vi "Individual curve visualization.vi"() -> ()   [LabVIEW 2020]
uses:
  <vilib>/Analysis/NI_AALPro.lvlib
panel:
  in  "parameter bounds":T1={"amp min"=-inf, "amp max"=inf, "power min"=-inf, "power max"=inf, "offset min"=0.0, "offset max"=0.0}
  out "residue":dbl
  out "amplitude":dbl
  out "Fitoffset":dbl
  out "power":dbl
  in  "Tab Control":enum32{"Drag R and 4T R", " Line cut"}(tab)=enum." Line cut"
  in  "Input figure":cluster{dbl[], dbl[]}[](graph)
  out "Mean vs Curve":cluster{dbl[], dbl[]}(graph)
  in  "Group #":i32=40
  out "Power vs Cursorx":cluster{dbl[], dbl[]}(graph)
  out "Waveform Chart":T2(graph)={"Cursor.Cursor Y"=229.6975806451613, "Cursor.Cursor X"=-46.37419354838706}
  in  "Drag V from V2":dbl[][](graph)=array2400x360[864000 elements]
  out "Vcut":cluster{dbl[], "Best Power Fit":dbl[]}[](graph)
  out "Idrive":cluster{dbl[], dbl[]}[](graph)
  out "Residue of T vs Cursorx":cluster{dbl[], dbl[]}(graph)
  in  "stop":bool
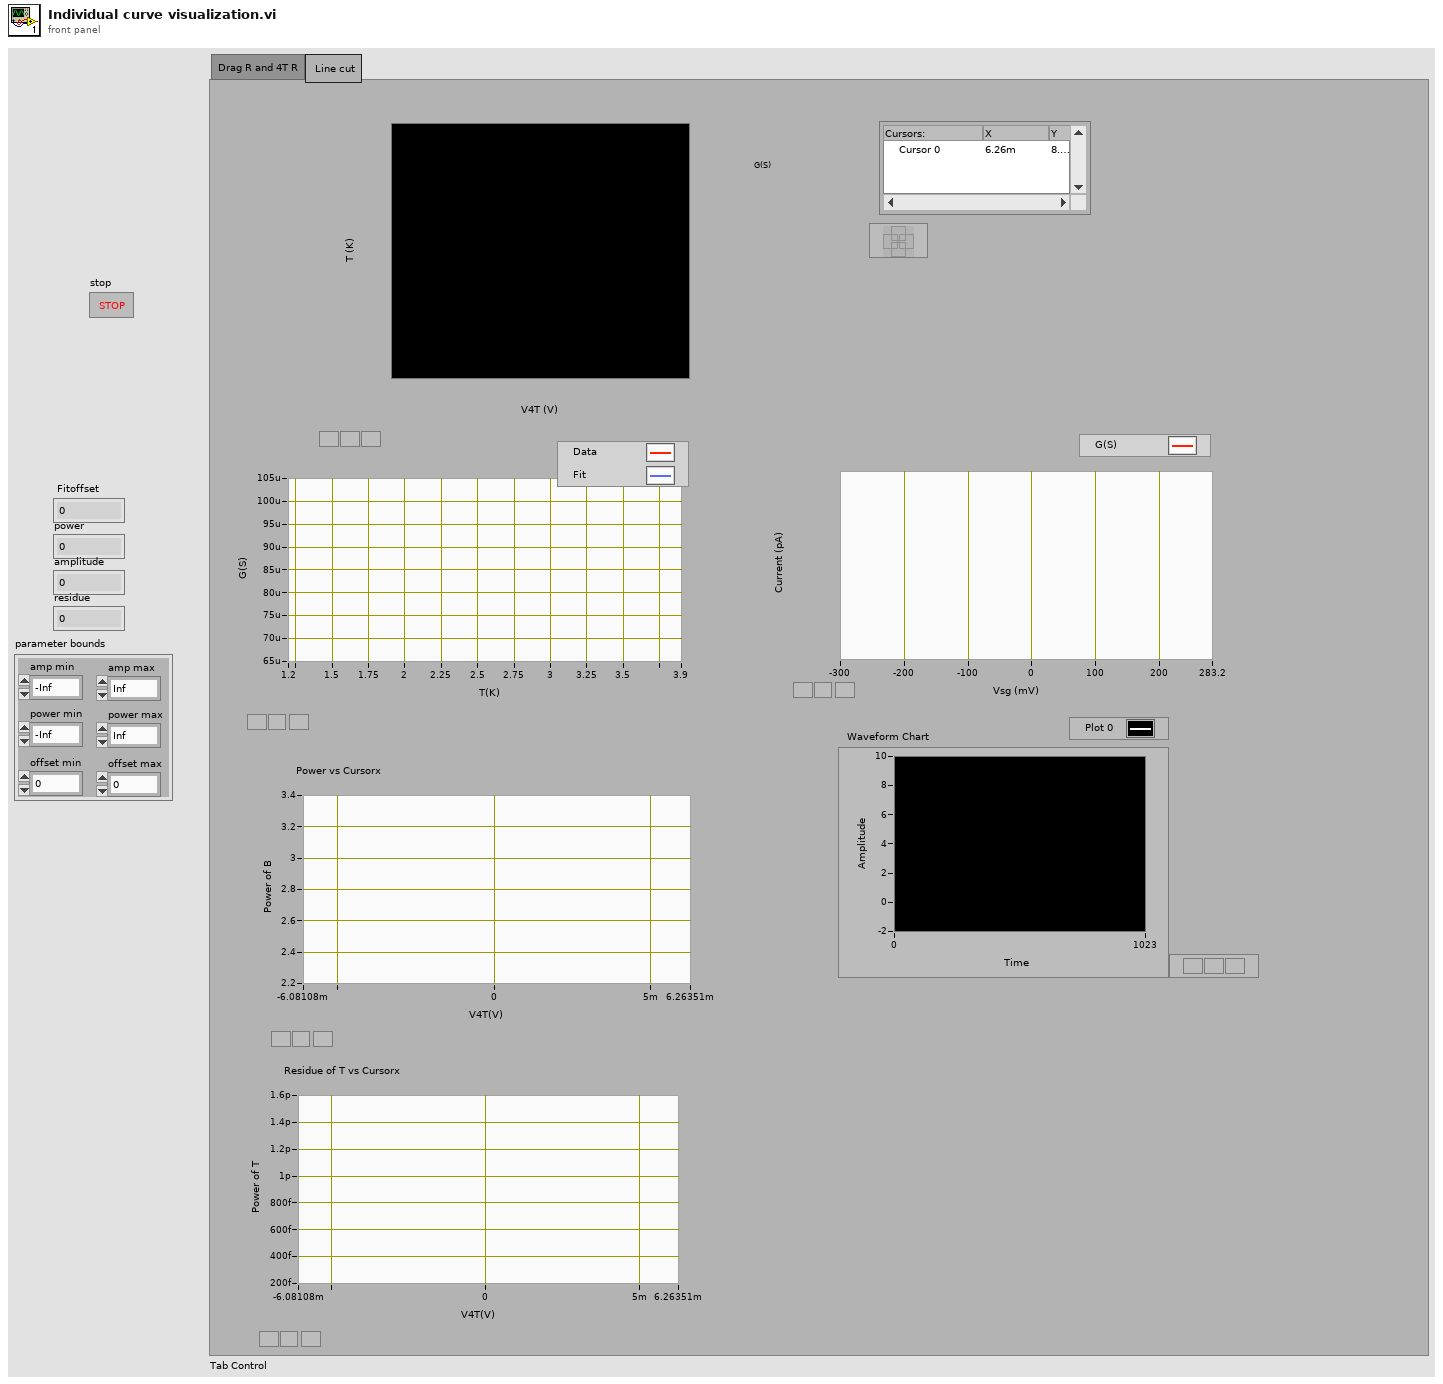
[diagram p1: front panel]
types:
  T1 = cluster{"amp min":dbl, "amp max":dbl, "power min":dbl, "power max":dbl, "offset min":dbl, "offset max":dbl}
  T2 = cluster{"Cursor.Cursor Y":dbl, "Cursor.Cursor X":dbl}
  T3 = typedef "LVOffsetAndMultiplierTypeDef.ctl" = cluster{"Offset":dbl, "Multiplier":dbl}
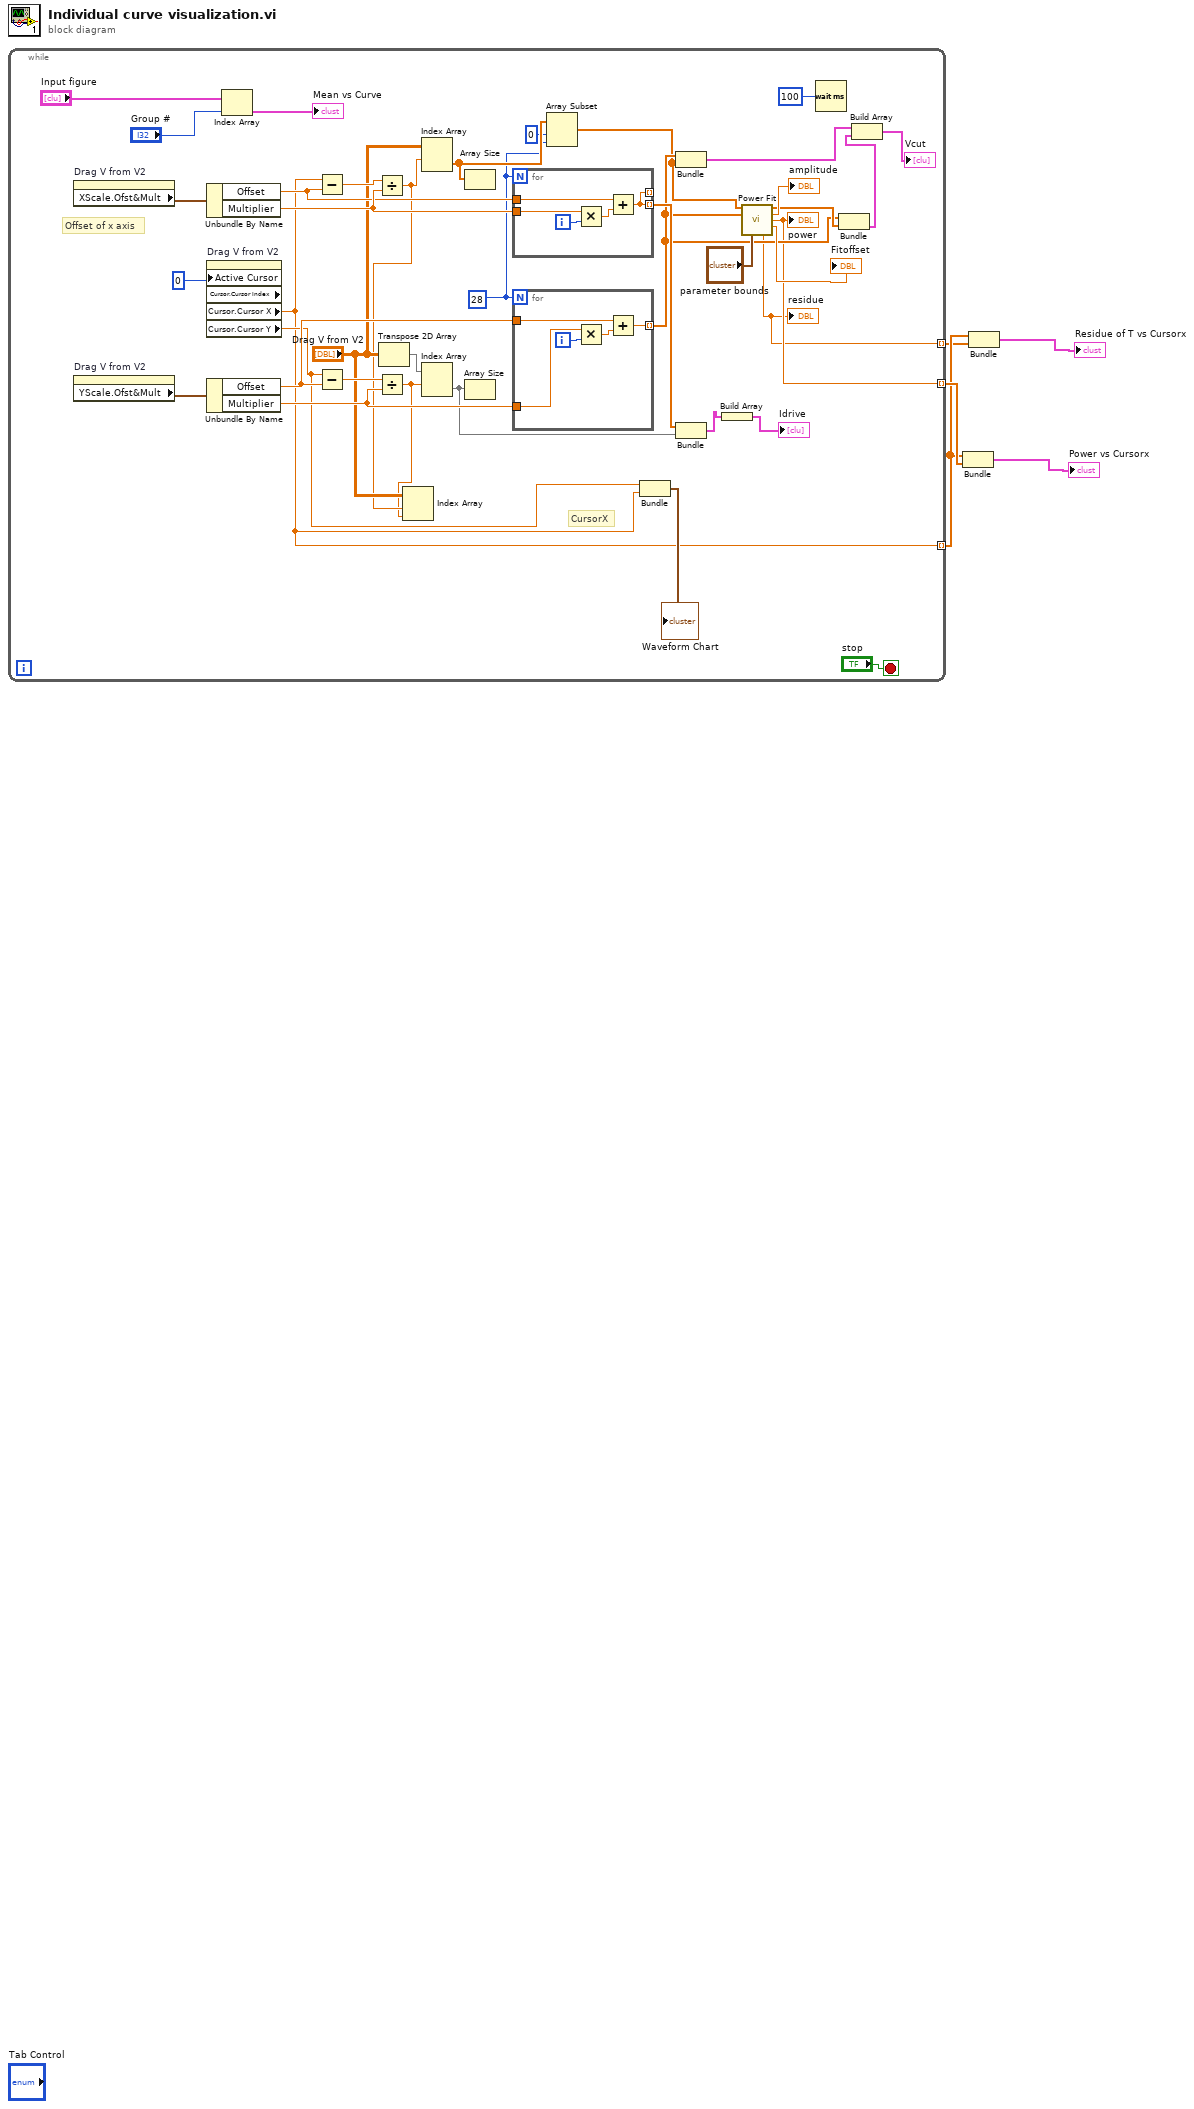
[diagram p0: block diagram]
diagram:
  n1 = while {
    tunnel: [w22] -> w2 mode=indexing
    tunnel: [w11] -> w4 mode=indexing
    tunnel: [w10] -> w1 mode=indexing
    stop <- "stop" stop-if-true
    w6 = 28
    # "CursorX"
    # "Offset of x axis"
    n2 = property on="Drag V from V2" class="IntGraph (strict)"() -> ("XScale.Ofst&Mult"=w37:T3)  [unwired: 2 in, 2 out]
    n3 = property on="Drag V from V2" class="IntGraph (strict)"() -> ("YScale.Ofst&Mult"=w39:T3)  [unwired: 2 in, 2 out]
    n4 = Unbundle By Name(w37) -> ("Offset"=w31:dbl, "Multiplier"=w32:dbl)
    n5 = property on="Drag V from V2" class="IntGraph (strict)" props=["Active Cursor", "Cursor", "Cursor Index", "Cursor", "Cursor X", "Cursor", "Cursor Y"]("Active Cursor"=u32 0) -> ("Cursor.Cursor X"=w22:dbl, "Cursor.Cursor Y"=w23:dbl)  [unwired: 2 in, 3 out]
    n6 = Unbundle By Name(w39) -> ("Offset"=w34:dbl, "Multiplier"=w35:dbl)
    n7 = Index Array(array="Input figure", index="Group #") -> (element=→"Mean vs Curve":cluster{dbl[], dbl[]})
    n8 = Subtract(x=w22, y=w31) -> (x-y=w36:dbl)
    n9 = Subtract(x=w23, y=w34) -> (x-y=w38:dbl)
    n10 = Divide(x=w36, y=w32) -> (x/y=w27:dbl)
    n11 = Divide(x=w38, y=w35) -> (x/y=w26:dbl)
    n12 = Transpose 2D Array(2D array="Drag V from V2") -> (transposed array=w41:dbl[][])
    n13 = Index Array(array="Drag V from V2", index (row)=w27, index (col)=w26) -> ()  [unwired: 1 out]
    n14 = Index Array(array="Drag V from V2", index (row)=w27) -> (element=w9:dbl[])  [unwired: 1 in]
    n15 = Index Array(array=w41, index (row)=w26) -> (element=w33:dbl[])  [unwired: 1 in]
    n16 = Array Size(array=w9) -> ()  [unwired: 1 out]
    n17 = Array Size(array=w33) -> ()  [unwired: 1 out]
    n18 = for {
      N: w6 -> [_]
      tunnel: w32 -> [w48]
      tunnel: w31 -> [w46]
      tunnel: [w45] -> _ mode=indexing
      tunnel: [w45] -> w30 mode=indexing
      i -> [w49]
      n19 = Multiply(x=w48, y=w49) -> (x*y=w47:dbl)
      n20 = Add(x=w46, y=w47) -> (x+y=w45:dbl)
    }
    n21 = for {
      N: w6 -> [_]
      tunnel: w35 -> [w53]
      tunnel: w34 -> [w51]
      tunnel: [w50] -> w15 mode=indexing
      i -> [w54]
      n22 = Multiply(x=w53, y=w54) -> (x*y=w52:dbl)
      n23 = Add(x=w51, y=w52) -> (x+y=w50:dbl)
    }
    n24 = Array Subset(array=w9, index=0, length=w6) -> (w8:dbl[])
    n25 = Bundle("Cursor.Cursor Y"=w23, "Cursor.Cursor X"=w22) -> (→"Waveform Chart":T2)  [unwired: 1 in]
    n26 = Bundle(w15, w8) -> (w13:cluster{dbl[], dbl[]})  [unwired: 1 in]
    n27 = Bundle(w30, w33) -> (w21:cluster{dbl[], dbl[]})  [unwired: 1 in]
    n28 = Build Array(w21) -> (→"Idrive":cluster{dbl[], dbl[]}[])
    n29 = call <vilib>:"Power Fit.vi"("Y"=w8, "X"=w15, "parameter bounds"="parameter bounds") -> ("Best Power Fit"=w16:dbl[], "amplitude"=→"amplitude":dbl, "power"=w11:dbl, "offset"=→"Fitoffset":dbl, "residue"=w10:dbl)  [unwired: 7 in, 1 out]
    "power" <- w11
    "residue" <- w10
    n30 = Wait (ms)(milliseconds to wait=u32 100) -> ()  [unwired: 1 out]
    n31 = Bundle(w15, "Best Power Fit"=w16) -> (w14:cluster{dbl[], "Best Power Fit":dbl[]})  [unwired: 1 in]
    n32 = Build Array(w13, w14) -> (→"Vcut":cluster{dbl[], "Best Power Fit":dbl[]}[])
  }
  n33 = Bundle(w2, w4) -> (→"Power vs Cursorx":cluster{dbl[], dbl[]})  [unwired: 1 in]
  n34 = Bundle(w2, w1) -> (→"Residue of T vs Cursorx":cluster{dbl[], dbl[]})  [unwired: 1 in]
